vi "ElevatorTest.vi"(0 "MotorControlDevRef":T1={"DeviceStatus"={"status"=FALSE, "code"=0, "source"=""}, "Type"=enum."PWM", "PWM"={"PWM Channel"=enum."Invalid", "DeadBand"={"Name"="", "maxPositivePwm"=0, "minPositivePwm"=0, "centerPwm"=0, "maxNegativePwm"=0, "minNegativePwm"=0, "angularRange"=0}}, "CAN"={"Device Number"=0, "Control Mode"=enum."Percent VBus", "Semaphore"=refnum, "Max Vout"=12.0, "TalonSRX Control Mode"=enum."Percent VBus"}, "Invert"=FALSE}, 1 "EncoderDevRef":T8={"DevStatus"={"status"=FALSE, "code"=0, "source"=""}, "EncoderIndex"=enum."Invalid", "CounterIndex"=enum."Ctr 1", "DistancePerCount"=2.0, "Decoding Type"=enum."4x"}, 2 "PID gains":T12={"proportional gain (Kc)"=1.0, "integral time (Ti, min)"=0.01, "derivative time (Td, min)"=0.0} {"derivative time (Td, min)" format="%.3f"; "integral time (Ti, min)" format="%.3f"; "proportional gain (Kc)" format="%.3f"}, 3 "Upper":bool, 4 "Manual":bool, 5 "Lower":bool, 6 "Upper Limit":dbl, 7 "Lower Limit":dbl, 11 "Override Pilot":bool, 17 "Override CoPilot":bool) -> ()   [LabVIEW 2015]
uses:
  <vilib>/Rock Robotics/WPI/Encoder/WPI_EncoderDevRef.ctl
  <vilib>/Rock Robotics/SystemInterfaces/Encoder/FPGA_EncoderIdx.ctl
  <vilib>/Rock Robotics/SystemInterfaces/Counter/FPGA_CounterCtrSystemIndex.ctl
  <vilib>/Rock Robotics/WPI/Encoder/WPI_EncoderType.ctl
  <vilib>/Rock Robotics/WPI/MotorControl/WPI_MotorControlDeviceRef.ctl
  <vilib>/Rock Robotics/WPI/MotorControl/WPI_MotorControlType.ctl
  <vilib>/Rock Robotics/SystemInterfaces/DIO/FPGA_DIOPWMChannel.ctl
  <vilib>/Rock Robotics/WPI/PWM/WPI_PWMDeadband.ctl
  <vilib>/Rock Robotics/WPI/CAN/Jaguar/SubVIs/WPI_CANJaguar_ControlMode.ctl
  <vilib>/Rock Robotics/WPI/CAN/TalonSRX/WPI_CANTalonSRX_APIControlMode.ctl
  <vilib>/addons/control/pid/pid.llb/PID (DBL).vi
  <vilib>/addons/control/pid/NI_PID_pid.lvlib
panel:
  in  "Encoder Distance":dbl
  out "Motor Set":dbl
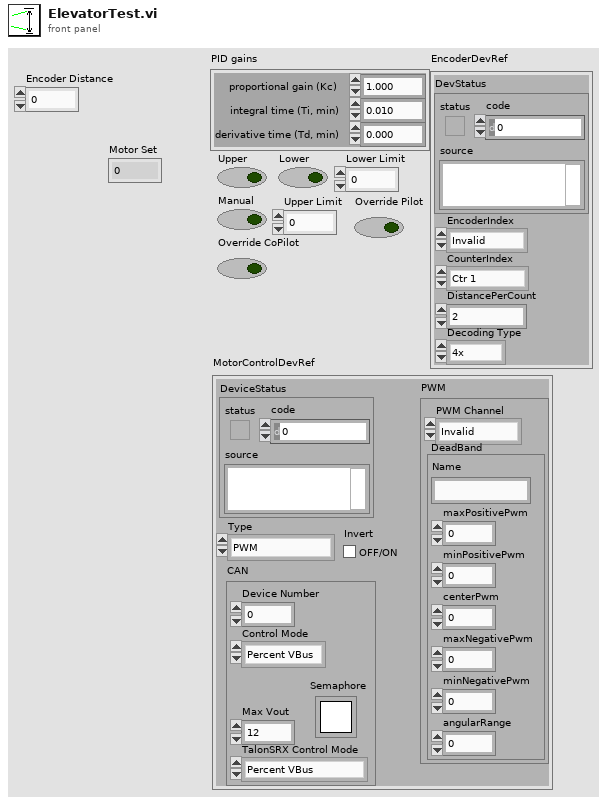
[diagram p1: front panel]
types:
  T1 = typedef "WPI_MotorControlDeviceRef.ctl" = cluster{"DeviceStatus":errorcluster, "Type":T2, "PWM":cluster{"PWM Channel":T3, "DeadBand":T4}, "CAN":cluster{"Device Number":u8, "Control Mode":T5, "Semaphore":T6, "Max Vout":dbl, "TalonSRX Control Mode":T7}, "Invert":bool}
  T2 = typedef "WPI_MotorControlType.ctl" = enum16{"PWM", "CAN", "CANTalonSRX"}
  T3 = typedef "FPGA_DIOPWMChannel.ctl" = enum8{"PWM 0", "PWM 1", "PWM 2", "PWM 3", "PWM 4", "PWM 5", "PWM 6", "PWM 7", "PWM 8", "PWM 9", "PWM MXP 0", "PWM MXP 1", "PWM MXP 2", "PWM MXP 3", "PWM MXP 4", "PWM MXP 5", "PWM MXP 6", "PWM MXP 7", "PWM MXP 8", "PWM MXP 9", "Invalid"}
  T4 = typedef "WPI_PWMDeadband.ctl" = cluster{"Name":string, "maxPositivePwm":i32, "minPositivePwm":i32, "centerPwm":i32, "maxNegativePwm":i32, "minNegativePwm":i32, "angularRange":u16}
  T5 = typedef "WPI_CANJaguar_ControlMode.ctl" = enum8{"Percent VBus", "Current", "Speed", "Position", "Voltage"}
  T6 = typedef "Semaphore RefNum" = refnum<k1>
  T7 = typedef "WPI_CANTalonSRX_APIControlMode.ctl" = enum8{"Percent VBus", "Speed", "Position", "Slave", "Unchanged / Invalid", "Voltage Compensation", "Current", "Motion Profile"}
  T8 = typedef "WPI_EncoderDevRef.ctl" = cluster{"DevStatus":errorcluster, "EncoderIndex":T9, "CounterIndex":T10, "DistancePerCount":dbl, "Decoding Type":T11}
  T9 = typedef "FPGA_EncoderIdx.ctl" = enum8{"Enc 0", "Enc 1", "Enc 2", "Enc 3", "Enc 4", "Enc 5", "Enc 6", "Enc 7", "Invalid"}
  T10 = typedef "FPGA_CounterCtrSystemIndex.ctl" = enum8{"Ctr 0", "Ctr 1", "Ctr 2", "Ctr 3", "Ctr 4", "Ctr 5", "Ctr 6", "Ctr 7", "Invalid"}
  T11 = typedef "WPI_EncoderType.ctl" = enum16{"1x", "2x", "4x"}
  T12 = cluster{"proportional gain (Kc)":dbl, "integral time (Ti, min)":dbl, "derivative time (Td, min)":dbl}
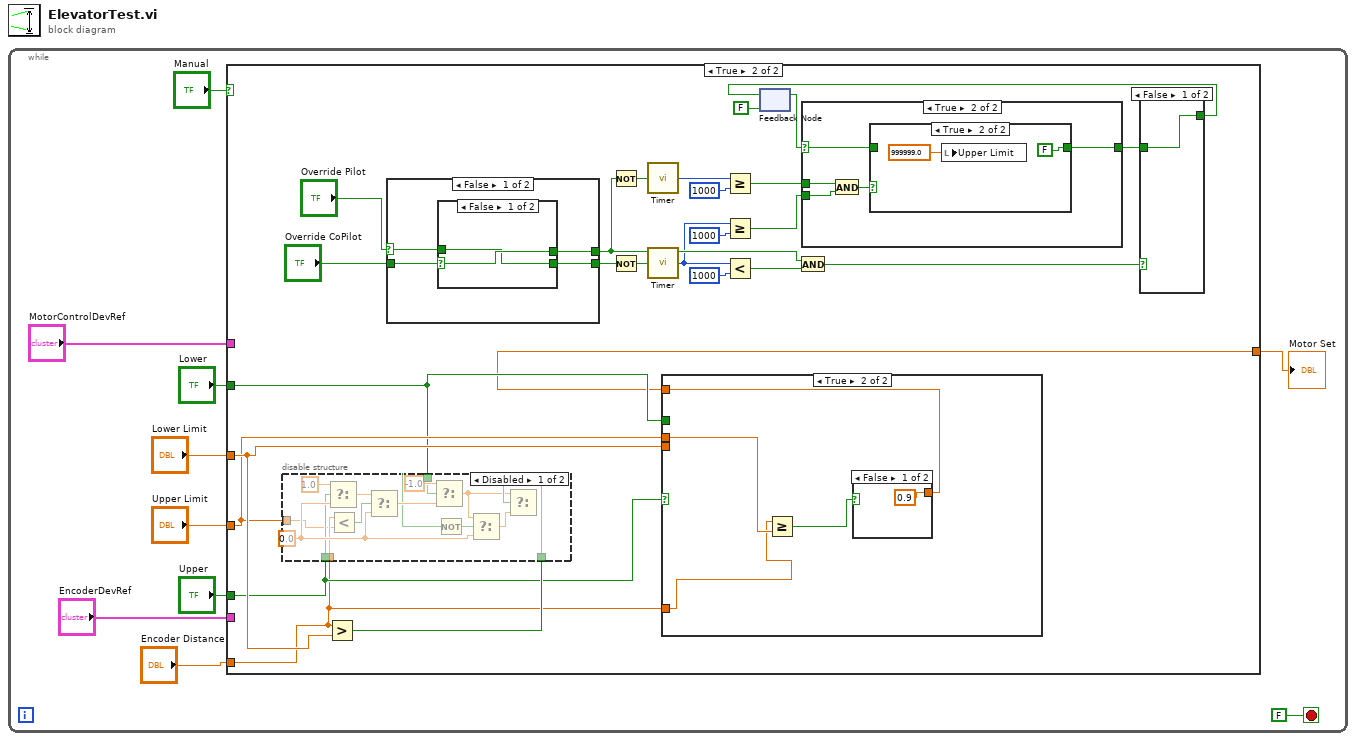
[diagram p0: block diagram]
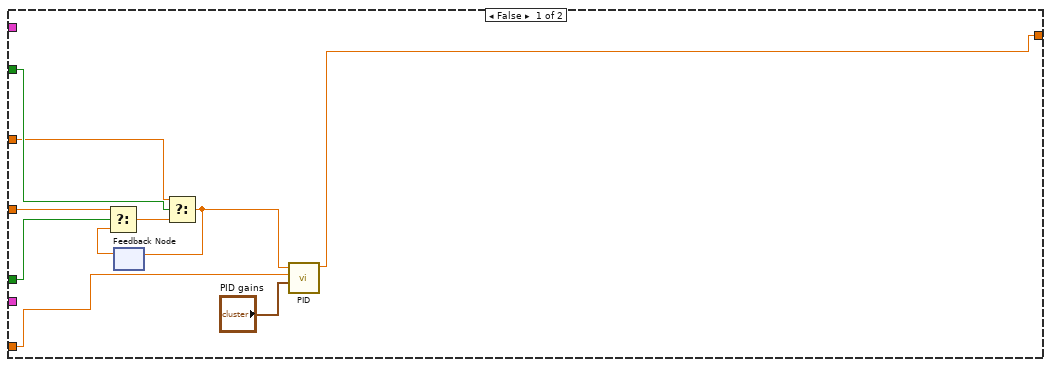
[diagram p2: hidden frame]
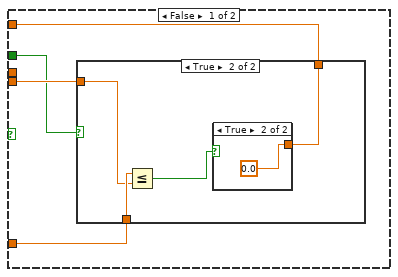
[diagram p4: hidden frame]
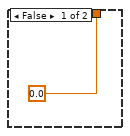
[diagram p5: hidden frame]
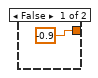
[diagram p6: hidden frame]
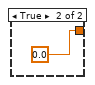
[diagram p7: hidden frame]
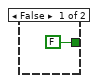
[diagram p8: hidden frame]
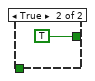
[diagram p10: hidden frame]
diagram:
  n1 = while {
    stop <- FALSE stop-if-true
    n2 = case shown="True" "Manual" {
      tunnel: "Upper" -> [w16 w23]
      tunnel: "Lower" -> [w15 w24]
      tunnel: "MotorControlDevRef" -> [_ _]
      tunnel: "EncoderDevRef" -> [_ _]
      tunnel: "Upper Limit" -> [w14 w25]
      tunnel: "Lower Limit" -> [w13 w26]
      tunnel: [w12 w22] -> w2
      tunnel: "Encoder Distance" -> [w11 w21]
      frame False {
        n3 = feedback #1() -> (w17:dbl)  [unwired: 1 in]
        n4 = Select(t=w14, s=w16, f=w17) -> (s? t:f=w19:dbl)
        n5 = Select(t=w13, s=w15, f=w19) -> (s? t:f=w18:dbl)
        n6 = feedback-in #1(w18) -> ()
        n7 = call-poly <vilib>:"PID.vi"("PID gains"="PID gains", "process variable"=w11, "setpoint"=w18) -> ("output"=w12:dbl)  [unwired: 7 in, 1 out]
      }
      frame True {
        n8 = Greater?(x=w21, y=w26) -> (0:w27:bool)
        n9 = disable-structure shown="Disabled" {
          disable-tunnel: w27 -> [w55 _]
          disable-tunnel: w21 -> [w50 _]
          disable-tunnel: w23 -> [w49 _]
          disable-tunnel: w24 -> [w48 _]
          disable-tunnel: w25 -> [w47 _]
          frame Disabled {
            w53 = 0.0 ("f")
            n10 = Select(t=1.0, s=w49, f=w53) -> (s? t:f=w58:dbl)
            n11 = Less?(x=w50, y=w47) -> (x < y?=w59:bool)
            n12 = Select(t=w58, s=w59, f=w53) -> (s? t:f=w57:dbl)
            n13 = Select(t=-1.0, s=w48, f=w57) -> (s? t:f=w52:dbl)
            n14 = Not(x=w48) -> (.not. x?=w51:bool)
            n15 = Select(t=w52, s=w51, f=w53) -> (s? t:f=w54:dbl)
            n16 = Select(t=w52, s=w55, f=w54) -> ()  [unwired: 1 out]
          }
          frame Enabled {
          }
        }
        n17 = case shown="False" "Override Pilot" {
          selector: "Override Pilot" -> [w89 w98]
          tunnel: "Override CoPilot" -> [w92 w97]
          tunnel: [w91 w97] -> w39
          tunnel: [w90 w98] -> w34
          frame False {
            n18 = case shown="False" w92 {
              selector: w92 -> [w94 w96]
              tunnel: [w94 w95] -> w91
              tunnel: [w93 w96] -> w90
              tunnel: w89 -> [w93 w95]
              frame False {
              }
              frame True {
              }
            }
          }
          frame True {
          }
        }
        n19 = Not(x=w39) -> (.not. x?=w37:bool)
        n20 = Not(x=w34) -> (.not. x?=w28:bool)
        n21 = call "Timer.vi"("Start Timer"=w37) -> ("Time elapsed"=w38:u64)
        n22 = call "Timer.vi"("Start Timer"=w28) -> ("Time elapsed"=w31:u64)
        n23 = case shown="True" w23 {
          tunnel: w21 -> [w64 w73]
          tunnel: w26 -> [w63 _]
          tunnel: [w62 w72] -> w22
          tunnel: w25 -> [_ w74]
          tunnel: w24 -> [w61 _]
          frame False {
            n24 = case shown="True" w61 {
              tunnel: w64 -> [_ w69]
              tunnel: w63 -> [_ w68]
              tunnel: [0.0 ("f") w66] -> w62
              frame False {
              }
              frame True {
                n25 = Less Or Equal?(x=w69, y=w68) -> (x <= y?=w67:bool)
                n26 = case shown="True" w67 {
                  tunnel: [-0.9 ("f") 0.0 ("f")] -> w66
                  frame False {
                  }
                  frame True {
                  }
                }
              }
            }
          }
          frame True {
            n27 = Greater Or Equal?(x=w73, y=w74) -> (x >= y?=w75:bool)
            n28 = case shown="False" w75 {
              tunnel: [0.9 ("f") 0.0 ("f")] -> w72
              frame False {
              }
              frame True {
              }
            }
          }
        }
        n29 = Greater Or Equal?(x=w38, y=u64 1000) -> (x >= y?=w44:bool)
        n30 = Greater Or Equal?(x=w31, y=u64 1000) -> (x >= y?=w43:bool)
        n31 = Less?(x=w31, y=u64 1000) -> (x < y?=w30:bool)
        n32 = feedback #2(FALSE) -> (w41:bool)
        n33 = And(x=w39, y=w30) -> (x .and. y?=w35:bool)
        n34 = case shown="True" w41 {
          selector: w41 -> [_ w79]
          tunnel: [FALSE w83] -> w42
          tunnel: w43 -> [_ w82]
          tunnel: w44 -> [_ w81]
          frame False {
          }
          frame True {
            n35 = And(x=w81, y=w82) -> (x .and. y?=w80:bool)
            n36 = case shown="True" w80 {
              tunnel: [w84 FALSE] -> w83
              tunnel: w79 -> [w84 _]
              frame False {
              }
              frame True {
                n37 = local write "Upper Limit"(999999.0 ("Upper Limit")) -> ()
              }
            }
          }
        }
        n38 = case shown="False" w35 {
          tunnel: [w87 TRUE] -> w36
          tunnel: w42 -> [w87 _]
          frame False {
          }
          frame True {
          }
        }
        n39 = feedback-in #2(w36) -> ()
      }
    }
    "Motor Set" <- w2
  }
